vi "SmartMoveDebugID.vi"(3 "error in":errorcluster caption="error out", 4 "Target (empty=readonly)":string, 5 "VISA resource":refnum<visa-resource-name>) -> (0 "error out":errorcluster, 1 "Found":string, 2 "VISA resource":refnum<visa-resource-name>)   [LabVIEW 8.6]
doc: "If Target is empty the actual STOPID will be returned.\nError: -1073807339 probably not switched on!"
panel:
  out "Try":i32
  out "return":string
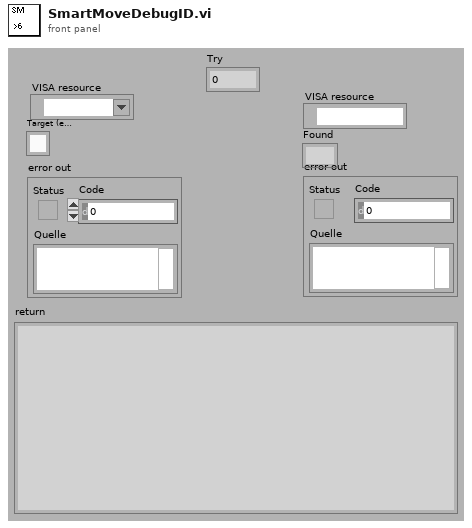
[diagram p1: front panel]
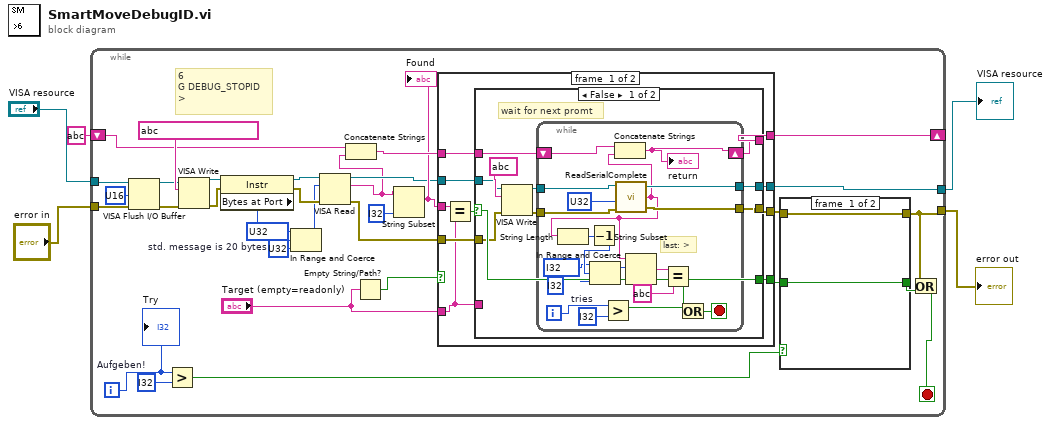
[diagram p0: block diagram]
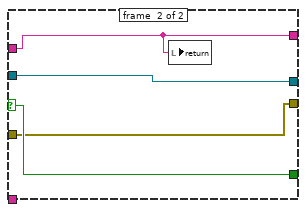
[diagram p2: hidden frame]
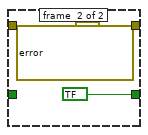
[diagram p4: hidden frame]
diagram:
  n1 = while {
    tunnel: "VISA resource" -> [w31]
    tunnel: "error in" -> [w29]
    tunnel: [w36] -> w4
    tunnel: [w6] -> w5
    shift-right: [w35] -> _
    shift-left: string ? ("read buffer") -> [w33]
    i -> [w27]
    stop <- w8 stop-if-true
    w13 = u32 ?  # std. message is 20 bytes
    w26 = i32 ?  # Aufgeben!
    # "6\nG DEBUG_STOPID\n>"
    n2 = VISA Flush I/O Buffer(VISA resource name=w31, mask (16)=u16 ? ("Maskieren (16)"), error in (no error)=w29) -> (VISA resource name out=w30:refnum<visa-resource-name>, error out=w28:errorcluster)
    n3 = Greater?(x=w27, y=w26) -> (0:w25:bool)
    n4 = VISA Write(VISA resource name=w30, write buffer=string ? ("Schreibpuffer"), error in (no error)=w28) -> (VISA resource name out=w21:refnum<visa-resource-name>, error out=w18:errorcluster)  [unwired: 1 out]
    n5 = property class="Instr"(reference=w21, error in=w18) -> (reference out=w20:refnum<visa-resource-name>, error out=w17:errorcluster, "Bytes at Port"=w15:u32)
    n6 = In Range and Coerce(upper limit=u32 ?, x=w15, lower limit=w13) -> (coerced(x)=w14:u32)  [unwired: 1 out]
    n7 = VISA Read(VISA resource name=w20, byte count=w14, error in (no error)=w17) -> (VISA resource name out=w19:refnum<visa-resource-name>, read buffer=w11:string, error out=w16:errorcluster)  [unwired: 1 out]
    n8 = Concatenate Strings(w33, w11) -> (w34:string)
    n9 = Empty String/Path?(string/path="Target (empty=readonly)") -> (empty?=w9:bool)
    n10 = String Subset(string=w11, length (rest)=i32 ? ("Länge (Rest)")) -> (substring=w22:string)  [unwired: 1 out]
    "Found" <- w22
    n11 = case shown="True" w9 {
      selector: w9 -> [_ w83]
      tunnel: [w47 w85] -> w36
      tunnel: [w46 w86] -> w35
      tunnel: w34 -> [w45 w86]
      tunnel: [w44 w84] -> w24
      tunnel: [w43 w83] -> w23
      tunnel: w22 -> [w42 _]
      tunnel: w19 -> [w41 w85]
      tunnel: w16 -> [w40 w84]
      tunnel: "Target (empty=readonly)" -> [w39 _]
      frame #0 {
        n12 = Equal?(x=w42, y=w39) -> (x = y?=w48:bool)
        n13 = case shown="False" w48 {
          selector: w48 -> [w55 w82]
          tunnel: [w55 w82] -> w43
          tunnel: [w54 w79] -> w47
          tunnel: [w53 w80] -> w44
          tunnel: [w52 w81] -> w46
          tunnel: w45 -> [w51 w81]
          tunnel: w39 -> [_ _]
          tunnel: w41 -> [w50 w79]
          tunnel: w40 -> [w49 w80]
          frame #0 {
            # "wait for next promt"
            n14 = VISA Write(VISA resource name=w50, write buffer=string ? ("Schreibpuffer"), error in (no error)=w49) -> (VISA resource name out=w57:refnum<visa-resource-name>, error out=w56:errorcluster)  [unwired: 1 out]
            n15 = while {
              tunnel: w57 -> [w71]
              tunnel: w56 -> [w70]
              tunnel: [w63] -> w54
              tunnel: [w62] -> w53
              shift-right: [w60] -> w52
              shift-left: w51 -> [w61]
              i -> [w67]
              stop <- w65 stop-if-true
              w66 = i32 ?  # tries
              # "last: >"
              n16 = Greater?(x=w67, y=w66) -> (0:w64:bool)
              n17 = call "ReadSerialComplete.vi"("error in"=w70, "milliseconds to wait"=u32 ? ("Zu wartende ms"), "duplicate VISA resource name"=w71) -> ("error out"=w62:errorcluster, "read buffer"=w59:string, "duplicate VISA resource name 2"=w63:refnum<visa-resource-name>)  [unwired: 1 in]
              n18 = String Length(string=w59) -> (length=w78:i32)
              n19 = Decrement(x=w78) -> (x-1=w76:i32)
              n20 = In Range and Coerce(upper limit=i32 ? ("oberer Grenzwert"), x=w76, lower limit=i32 ? ("unterer Grenzwert")) -> (coerced(x)=w77:i32)  [unwired: 1 out]
              n21 = Concatenate Strings(w61, w59) -> (w60:string)
              "return" <- w60
              n22 = String Subset(string=w59, offset (0)=w77) -> (substring=w75:string)  [unwired: 1 out]
              n23 = Equal?(x=w75, y=string ?) -> (x = y?=w73:bool)
              n24 = Or(x=w64, y=w73) -> (x .or. y?=w65:bool)
            }
          }
          frame #1 {
            n25 = local write "return"(w81) -> ()
          }
        }
      }
      frame #1 {
        # "empty input  get only"
      }
    }
    n26 = case shown="True" w25 {
      tunnel: w24 -> [w88 _]
      tunnel: [w88 errorcluster ? ("error out")] -> w6
      tunnel: w23 -> [w87 _]
      tunnel: [w87 bool ?] -> w7
      frame #0 {
      }
      frame #1 {
      }
    }
    n27 = Or(x=w6, y=w7) -> (x .or. y?=w8:bool)
    "Try" <- w27
  }
  "error out" <- w5
  "VISA resource" <- w4
